vi "DC Source Core Logic.vi"(8 "error in":errorcluster, 9 "measurement configuration":T1={"Pin Name"="Pin1", "Voltage Level (V)"=2.0, "Voltage Level Range (V)"=6.0, "Current Limit (A)"=0.01, "Current Limit Range (A)"=0.01, "Source Delay (s)"=0.1} {"Source Delay (s)" format="%#_6p"; "Current Limit Range (A)" format="%#_6p"; "Current Limit (A)" format="%#_6p"; "Voltage Level Range (V)" format="%#_6p"; "Voltage Level (V)" format="%#_6p"}, 10 "instrument handle":refnum<k15>, 11 "channel list":string) -> (0 "error out":errorcluster, 1 "in compliance?":bool, 2 "measured current":dbl, 3 "instrument handle out":refnum<k15>, 4 "calculated power":dbl, 5 "measured voltage":dbl)   [LabVIEW 2024, in "NIDCPowerPPS.lvlib"]
uses:
  NIDCPowerPPS.lvlib
  Measurement Configuration.ctl
  <instrlib>/niDCPower/nidcpower.llb/niDCPower Source Mode.ctl
  <instrlib>/niDCPower/nidcpower.llb/niDCPower Output Function.ctl
  <instrlib>/niDCPower/nidcpower.llb/niDCPower Wait For Event - Event.ctl
  <instrlib>/niDCPower/nidcpower.llb/niDCPower Measurement Type.ctl
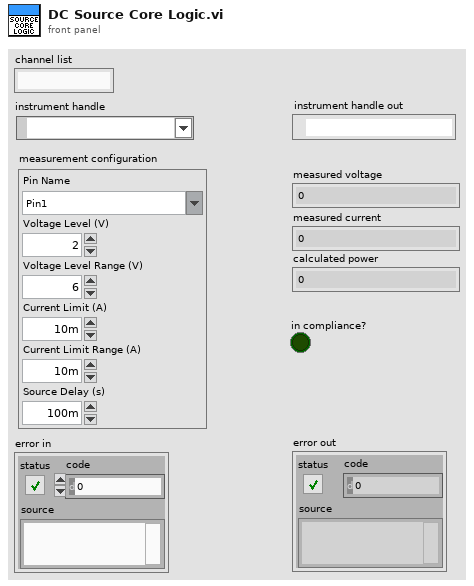
[diagram p1: front panel]
types:
  T1 = typedef "NIDCPowerPPS.lvlib/Measurement Configuration.ctl" = cluster{"Pin Name":string, "Voltage Level (V)":dbl, "Voltage Level Range (V)":dbl, "Current Limit (A)":dbl, "Current Limit Range (A)":dbl, "Source Delay (s)":dbl}
  T2 = typedef "niDCPower Measurement Type.ctl" = i32
  T3 = typedef "niDCPower Wait For Event - Event.ctl" = i32
  T4 = typedef "niDCPower Output Function.ctl" = i32
  T5 = typedef "niDCPower Source Mode.ctl" = i32
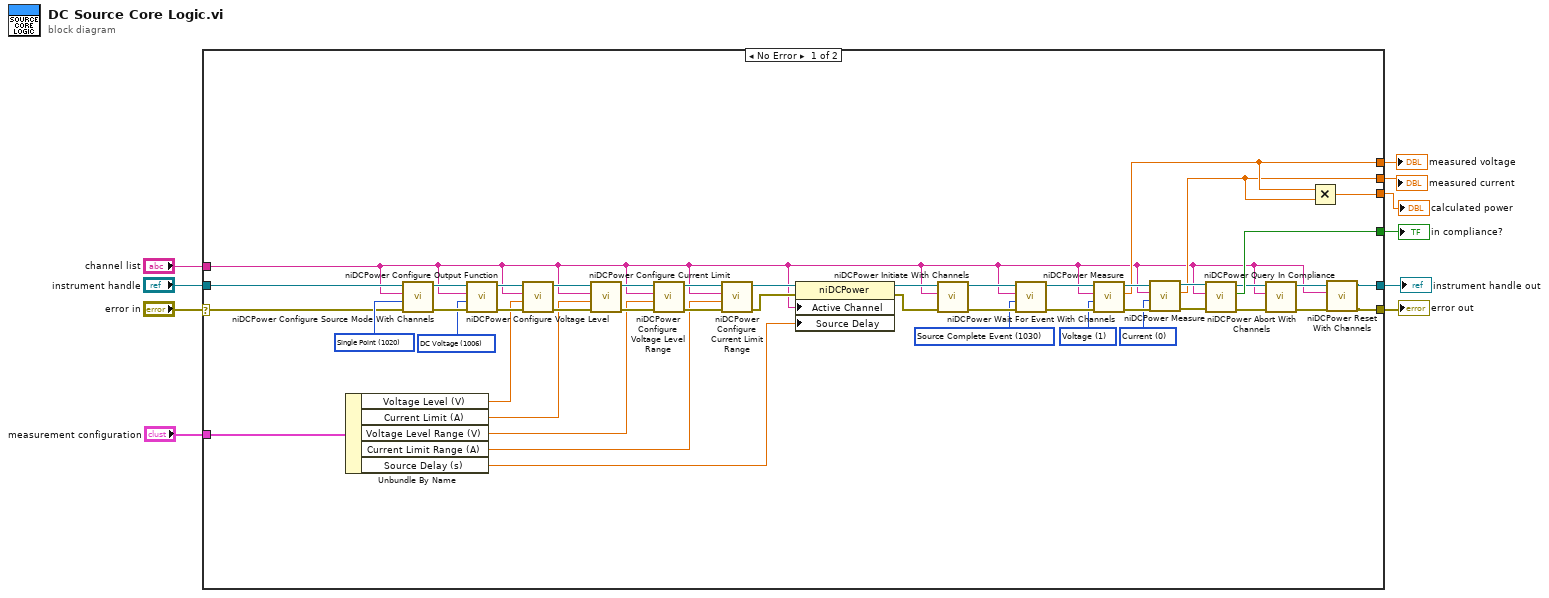
[diagram p0: block diagram]
diagram:
  n1 = case shown="No Error" "error in" {
    selector: "error in" -> [w31 w57]
    tunnel: [w12 w57] -> w10
    tunnel: "instrument handle" -> [w32 w58]
    tunnel: [w13 w58] -> w8
    tunnel: "channel list" -> [w11 _]
    tunnel: "measurement configuration" -> [w30 _]
    tunnel: [w21 _] -> w5
    tunnel: [w20 _] -> w4
    tunnel: [w19 _] -> w3
    tunnel: [w18 _] -> w2
    frame No Error {
      w22 = T2 0 items=["Current", "Voltage"] ("measurement type")
      w23 = T2 1 items=["Current", "Voltage"] ("measurement type")
      w36 = T3 1030 items=["Source Complete Event"=1030, "Measure Complete Event"=1031, "Sequence Iteration Complete Event"=1032, "Sequence Engine Done Event"=1033, "Pulse Complete Event"=1051, "Ready For Pulse Trigger Event"=1052] ("event")
      w39 = T4 1006 items=["DC Voltage"=1006, "DC Current"=1007, "Pulse Voltage"=1049, "Pulse Current"=1050] ("output function")
      w40 = T5 1020 items=["Single Point"=1020, "Sequence"=1021] ("source mode")
      n2 = Unbundle By Name(w30) -> ("Voltage Level (V)"=w38:dbl, "Current Limit (A)"=w37:dbl, "Voltage Level Range (V)"=w35:dbl, "Current Limit Range (A)"=w34:dbl, "Source Delay (s)"=w33:dbl)
      n3 = call <instrlib>:"niDCPower Configure Source Mode With Channels.vi"("error in (no error)"=w31, "source mode"=w40, "channel name"=w11, "instrument handle"=w32) -> ("error out"=w54:errorcluster, "instrument handle out"=w53:refnum<k15>)  [unwired: 6 in]
      n4 = call <instrlib>:"niDCPower Configure Output Function.vi"("error in (no error)"=w54, "output function"=w39, "channel name"=w11, "instrument handle"=w53) -> ("error out"=w41:errorcluster, "instrument handle out"=w42:refnum<k15>)  [unwired: 6 out]
      n5 = call <instrlib>:"niDCPower Configure Voltage Level.vi"("error in (no error)"=w41, "voltage level"=w38, "channel name"=w11, "instrument handle"=w42) -> ("error out"=w55:errorcluster, "instrument handle out"=w56:refnum<k15>)  [unwired: 6 out]
      n6 = call <instrlib>:"niDCPower Configure Current Limit.vi"("error in (no error)"=w55, "current limit"=w37, "channel name"=w11, "instrument handle"=w56) -> ("error out"=w52:errorcluster, "instrument handle out"=w51:refnum<k15>)  [unwired: 1 in, 5 out]
      n7 = call <instrlib>:"niDCPower Configure Voltage Level Range.vi"("error in (no error)"=w52, "voltage level range"=w35, "channel name"=w11, "instrument handle"=w51) -> ("error out"=w50:errorcluster, "instrument handle out"=w49:refnum<k15>)  [unwired: 6 out]
      n8 = call <instrlib>:"niDCPower Configure Current Limit Range.vi"("error in (no error)"=w50, "current limit range"=w34, "channel name"=w11, "instrument handle"=w49) -> ("error out"=w45:errorcluster, "instrument handle out"=w48:refnum<k15>)  [unwired: 6 out]
      n9 = property class="niDCPower"(reference=w48, error in=w45, "Active Channel"=w11, "Source Delay"=w33) -> (reference out=w47:refnum<k15>, error out=w46:errorcluster)
      n10 = call <instrlib>:"niDCPower Initiate With Channels.vi"("error in (no error)"=w46, "channel name"=w11, "instrument handle"=w47) -> ("error out"=w43:errorcluster, "instrument handle out"=w44:refnum<k15>)  [unwired: 7 in]
      n11 = call <instrlib>:"niDCPower Wait For Event With Channels.vi"("error in (no error)"=w43, "event"=w36, "channel name"=w11, "instrument handle"=w44) -> ("error out"=w28:errorcluster, "instrument handle out"=w29:refnum<k15>)  [unwired: 6 in]
      n12 = call <instrlib>:"niDCPower Measure.vi"("error in (no error)"=w28, "measurement type"=w23, "channel name"=w11, "instrument handle"=w29) -> ("error out"=w25:errorcluster, "measurement"=w21:dbl, "instrument handle out"=w27:refnum<k15>)  [unwired: 5 in]
      n13 = call <instrlib>:"niDCPower Measure.vi"("error in (no error)"=w25, "measurement type"=w22, "channel name"=w11, "instrument handle"=w27) -> ("error out"=w24:errorcluster, "measurement"=w20:dbl, "instrument handle out"=w26:refnum<k15>)  [unwired: 5 in]
      n14 = call <instrlib>:"niDCPower Query In Compliance.vi"("error in (no error)"=w24, "channel name"=w11, "instrument handle"=w26) -> ("error out"=w16:errorcluster, "in compliance?"=w18:bool, "instrument handle out"=w17:refnum<k15>)  [unwired: 6 out]
      n15 = call <instrlib>:"niDCPower Abort With Channels.vi"("error in (no error)"=w16, "channel name"=w11, "instrument handle"=w17) -> ("error out"=w15:errorcluster, "instrument handle out"=w14:refnum<k15>)  [unwired: 7 in]
      n16 = Multiply(x=w21, y=w20) -> (x*y=w19:dbl)
      n17 = call <instrlib>:"niDCPower Reset With Channels.vi"("error in (no error)"=w15, "channel name"=w11, "instrument handle"=w14) -> ("error out"=w12:errorcluster, "instrument handle out"=w13:refnum<k15>)  [unwired: 7 in]
    }
    frame Error {
    }
  }
  "error out" <- w10
  "instrument handle out" <- w8
  "measured voltage" <- w5
  "measured current" <- w4
  "calculated power" <- w3
  "in compliance?" <- w2
